vi "TEST_MenuRTM.vi"(10 "Color Theme":enum16{"LabVIEW", "Dark", "Windows Gray"}(ring), 11 "ExitEvent":refnum<user-event>) -> ()   [LabVIEW 2021]
uses:
  Menu.lvclass
  Picture2D/src/Font/Font.lvclass
  Picture2D/src/Square/Square.lvclass
  C:/GitHub/Picture2D/src/Polygone/Polygone.lvclass
  C:/GitHub/Picture2D/src/Rectangle/Rectangle.lvclass
  C:/GitHub/Picture2D/src/Shape/Shape.lvclass
  C:/GitHub/Picture2D/src/Picture2D/Picture2D.lvclass
  Picture2D/src/Point/Point.lvclass
  Picture2D/src/Font/Font.lvclass/Font.ctl
  Picture2D/src/Color/Color.lvclass
  SubMenuIcon.ctl
  4d7882bf-4570-41b5-8159-e9b7f331f501.vi
  Picture2D/src/Font/SetFontName.vi
  Picture2D/src/Font/SetSize.vi
  SetBackgroundColor.vi
  SetBorderColor.vi
  SetHiliteColor.vi
  SetHiliteTextColor.vi
  SetTextColor.vi
  SetFont.vi
  SetDesiredFont.vi
  SetSubMenuIconType.vi
  SetSubMenuIconOpened.vi
  SetSubMenuIconClosed.vi
  <vilib>/ErrorRing/Error Ring.xnode
panel:
  out "2D Picture":picture
  in  "Font Name":string="Arial"
  in  "Size":i16=16
  in  "Desired Font":T1(ring)=enum."Application Font"
  out "ItemPath":string
  out "ItemTag":string
  out "error out":errorcluster
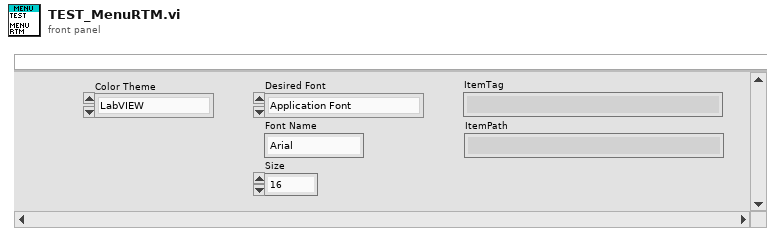
[diagram p1: front panel]
types:
  T1 = enum16{"User-specified Font", "Application Font", "System Font", "Dialog Font"}
  T2 = typedef "Menu.lvlib/Menu.lvclass/SubMenuIcon.ctl" = enum16{"LabVIEW", "Windows", "Custom"}
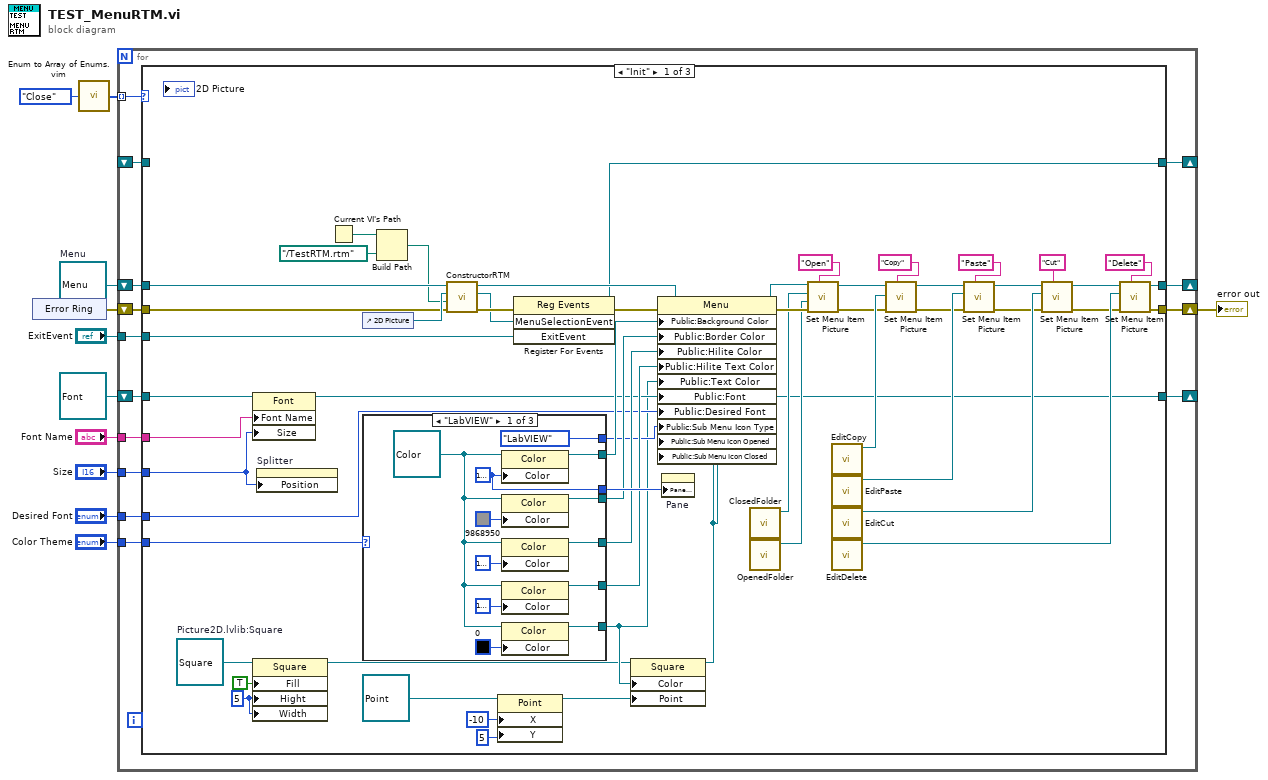
[diagram p0: block diagram]
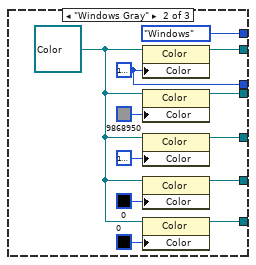
[diagram p2: hidden frame]
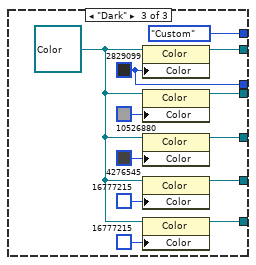
[diagram p3: hidden frame]
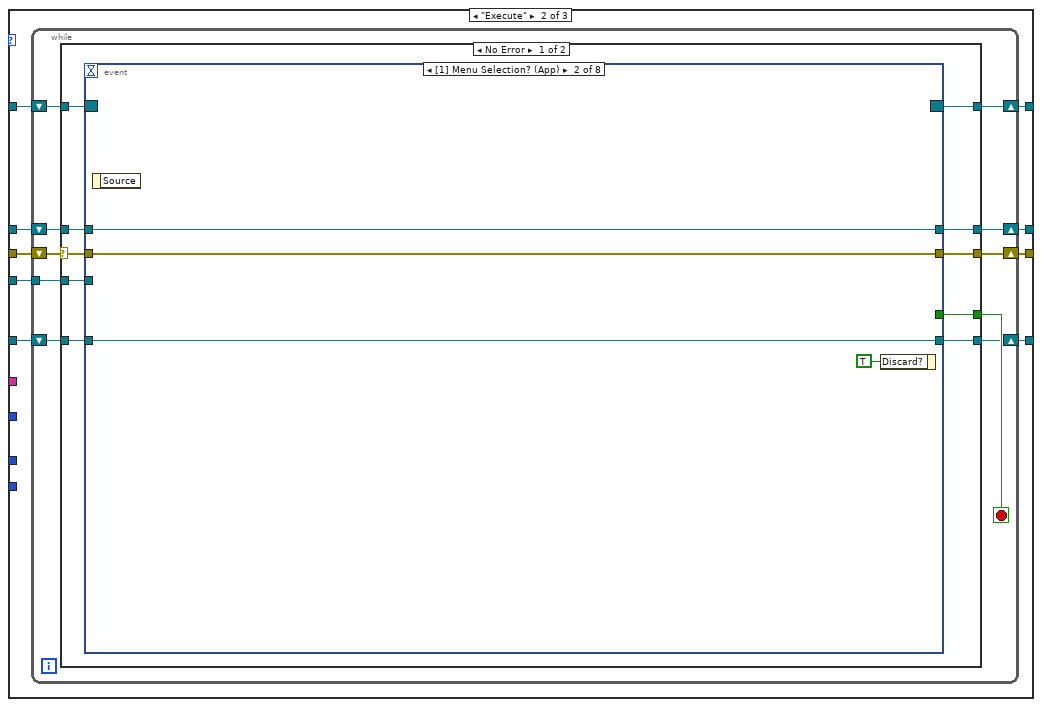
[diagram p4: hidden frame]
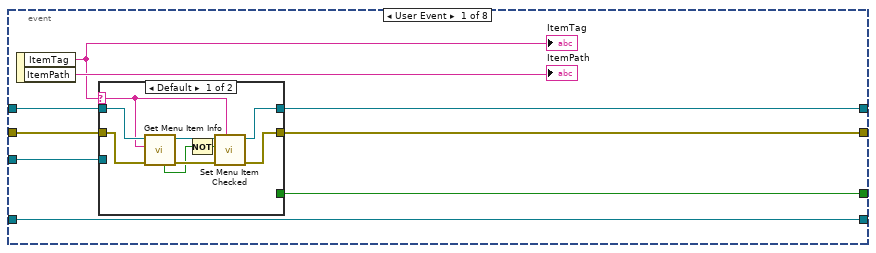
[diagram p5: hidden frame]
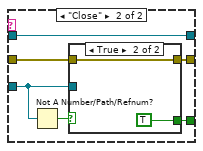
[diagram p6: hidden frame]
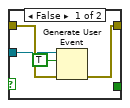
[diagram p7: hidden frame]
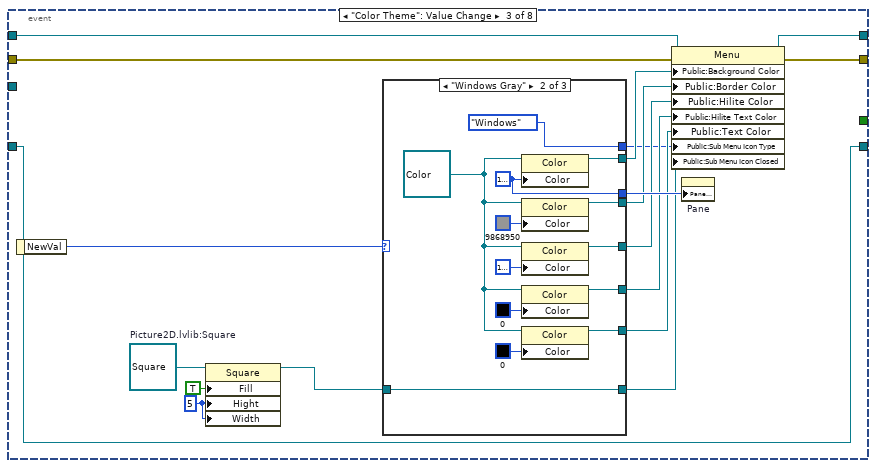
[diagram p8: hidden frame]
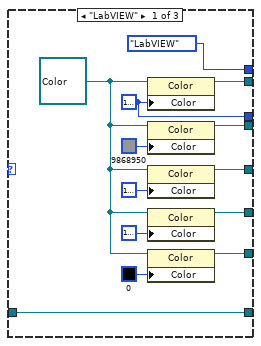
[diagram p9: hidden frame]
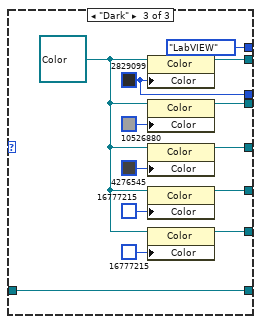
[diagram p10: hidden frame]
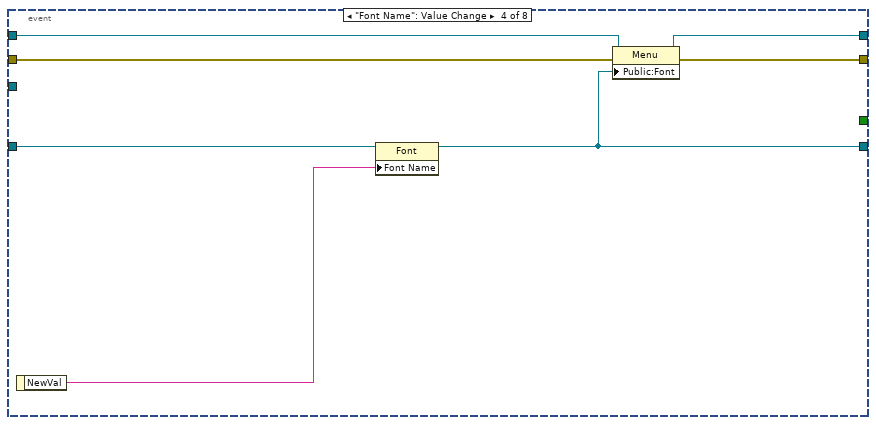
[diagram p11: hidden frame]
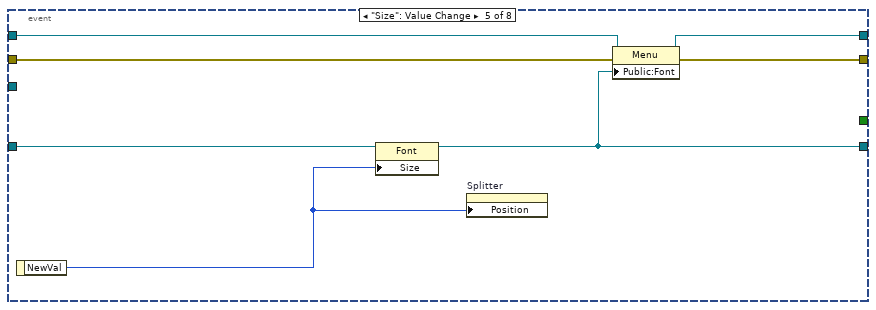
[diagram p12: hidden frame]
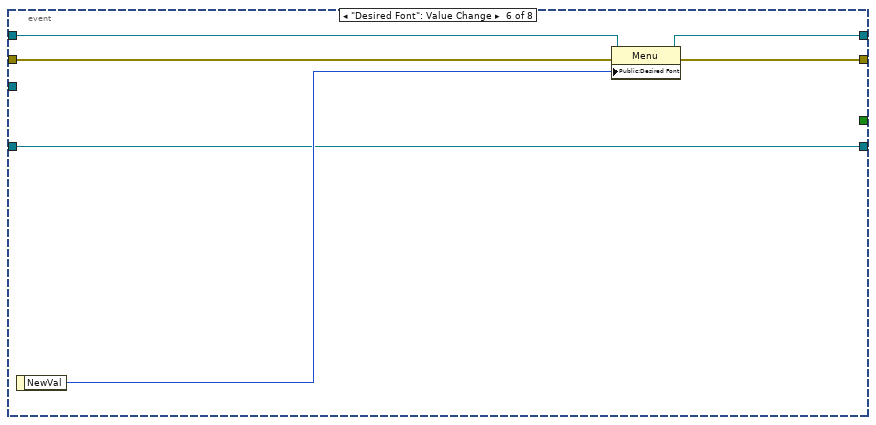
[diagram p13: hidden frame]
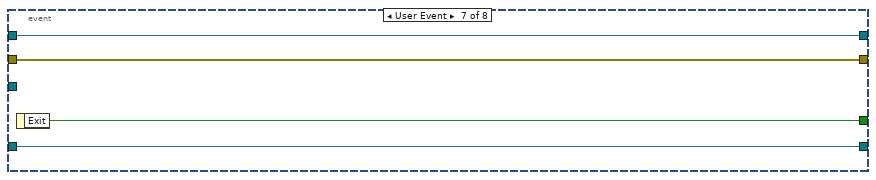
[diagram p14: hidden frame]
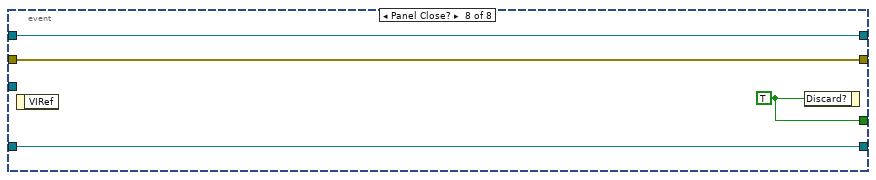
[diagram p15: hidden frame]
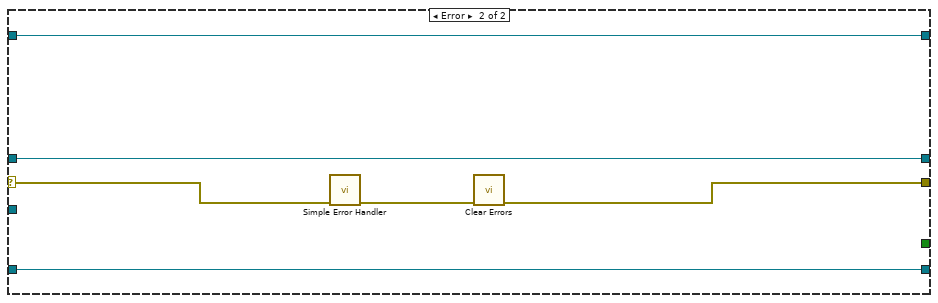
[diagram p16: hidden frame]
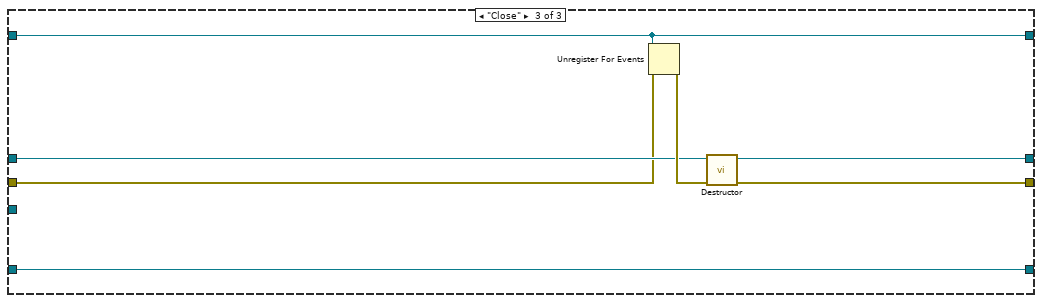
[diagram p17: hidden frame]
diagram:
  w3 = refnum<class "Menu.lvclass"> refnum  # Menu
  n1 = xnode "Error Ring"() -> ("error out"=w2:errorcluster)
  n2 = call "Enum to Array of Enums.vim"("enum"=enum16{"Init", "Execute", "Close"}."Close") -> ("array of enums"=w10:enum16{"Init", "Execute", "Close"}[])
  n3 = for {
    tunnel: "ExitEvent" -> [w22]
    shift-right: [w12] -> _
    shift-left: _ -> [w25]
    shift-right: [w14] -> w1
    shift-left: w2 -> [w24]
    shift-right: [w13] -> _
    shift-left: w3 -> [w23]
    tunnel: w10 -> [w21] mode=indexing
    tunnel: "Font Name" -> [w19]
    tunnel: "Size" -> [w18]
    tunnel: "Desired Font" -> [w17]
    tunnel: "Color Theme" -> [w16]
    shift-right: [w15] -> _
    shift-left: refnum<class "Font.lvclass"> refnum ("Fonts") -> [w20]
    n4 = case shown="\"Init\"" w21 {
      tunnel: w25 -> [_ w127 w274]
      tunnel: [w46 w126 w275] -> w13
      tunnel: [w44 w125 w274] -> w12
      tunnel: [w45 w124 w277] -> w14
      tunnel: w24 -> [w38 w123 w273]
      tunnel: w23 -> [w47 w122 w275]
      tunnel: w22 -> [w43 w121 _]
      tunnel: w20 -> [w56 w120 w276]
      tunnel: w19 -> [w55 _ _]
      tunnel: w18 -> [w37 _ _]
      tunnel: w17 -> [w54 _ _]
      tunnel: w16 -> [w48 _ _]
      tunnel: [w42 w119 w276] -> w15
      frame "Init" {
        w33 = i16 5 ("Hight")
        w35 = refnum<class "Square.lvclass"> refnum  # Picture2D.lvlib:Square
        n5 = property class="Font"(reference=w56, "Font Name"=w55, "Size"=w37) -> (reference out=w42:refnum<class "Font.lvclass">)  [unwired: 1 in, 1 out]
        n6 = property class="Square"(reference=w35, "Fill"=TRUE, "Hight"=w33, "Width"=w33) -> (reference out=w27:refnum<class "Square.lvclass">)  [unwired: 1 in, 1 out]
        n7 = property on="Splitter" class="Splitter"("Position"=w37) -> ()  [unwired: 2 in, 2 out]
        n8 = Current VI's Path() -> (path=w41:path)
        n9 = control-ref of="2D Picture"() -> (w60:refnum<vi>)
        n10 = case shown="\"LabVIEW\"" w48 {
          tunnel: [w94 w106 w118] -> w62
          tunnel: [w92 w104 w116] -> w63
          tunnel: [w91 w103 w115] -> w64
          tunnel: [w90 w102 w114] -> w65
          tunnel: [w89 w101 w113] -> w32
          tunnel: [w84 w96 w108] -> w66
          tunnel: [SubMenuIcon."LabVIEW" ("SubMenuIconType") SubMenuIcon."Windows" ("SubMenuIconType") SubMenuIcon."Custom" ("SubMenuIconType")] -> w36
          frame "LabVIEW" {
            w84 = u32 16777238 ("Color")
            w93 = refnum<class "Color.lvclass"> refnum ("Background Color")
            n11 = property class="Color"(reference=w93, "Color"=w84) -> (reference out=w94:refnum<class "Color.lvclass">)  [unwired: 1 in, 1 out]
            n12 = property class="Color"(reference=w93, "Color"=u32 9868950) -> (reference out=w92:refnum<class "Color.lvclass">)  [unwired: 1 in, 1 out]
            n13 = property class="Color"(reference=w93, "Color"=u32 16777224) -> (reference out=w91:refnum<class "Color.lvclass">)  [unwired: 1 in, 1 out]
            n14 = property class="Color"(reference=w93, "Color"=u32 16777226) -> (reference out=w90:refnum<class "Color.lvclass">)  [unwired: 1 in, 1 out]
            n15 = property class="Color"(reference=w93, "Color"=u32 0) -> (reference out=w89:refnum<class "Color.lvclass">)  [unwired: 1 in, 1 out]
          }
          frame "Windows Gray" {
            w96 = u32 16777238 ("Color")
            w105 = refnum<class "Color.lvclass"> refnum ("Background Color")
            n16 = property class="Color"(reference=w105, "Color"=w96) -> (reference out=w106:refnum<class "Color.lvclass">)  [unwired: 1 in, 1 out]
            n17 = property class="Color"(reference=w105, "Color"=u32 9868950) -> (reference out=w104:refnum<class "Color.lvclass">)  [unwired: 1 in, 1 out]
            n18 = property class="Color"(reference=w105, "Color"=u32 16777225) -> (reference out=w103:refnum<class "Color.lvclass">)  [unwired: 1 in, 1 out]
            n19 = property class="Color"(reference=w105, "Color"=u32 0) -> (reference out=w102:refnum<class "Color.lvclass">)  [unwired: 1 in, 1 out]
            n20 = property class="Color"(reference=w105, "Color"=u32 0) -> (reference out=w101:refnum<class "Color.lvclass">)  [unwired: 1 in, 1 out]
          }
          frame "Dark" {
            w108 = u32 2829099 ("Color")
            w117 = refnum<class "Color.lvclass"> refnum ("Background Color")
            n21 = property class="Color"(reference=w117, "Color"=w108) -> (reference out=w118:refnum<class "Color.lvclass">)  [unwired: 1 in, 1 out]
            n22 = property class="Color"(reference=w117, "Color"=u32 10526880) -> (reference out=w116:refnum<class "Color.lvclass">)  [unwired: 1 in, 1 out]
            n23 = property class="Color"(reference=w117, "Color"=u32 4276545) -> (reference out=w115:refnum<class "Color.lvclass">)  [unwired: 1 in, 1 out]
            n24 = property class="Color"(reference=w117, "Color"=u32 16777215) -> (reference out=w114:refnum<class "Color.lvclass">)  [unwired: 1 in, 1 out]
            n25 = property class="Color"(reference=w117, "Color"=u32 16777215) -> (reference out=w113:refnum<class "Color.lvclass">)  [unwired: 1 in, 1 out]
          }
        }
        n26 = Build Path(base path=w41, name or relative path=path "../TestRTM.rtm") -> (appended path=w39:path)
        n27 = call "ConstructorRTM.vi"("error in (no error)"=w38, "RTM Path"=w39, "PictRef"=w60, "Menu in"=w47) -> ("error out"=w59:errorcluster, "MenuSelectionEvent"=w57:refnum<user-event>, "Menu out"=w61:refnum<class "Menu.lvclass">)  [unwired: 5 in]
        n28 = property class="Point"(reference=refnum<class "Point.lvclass"> refnum ("Point"), "X"=i16 -10, "Y"=i16 5) -> (reference out=w30:refnum<class "Point.lvclass">)  [unwired: 1 in, 1 out]
        n29 = register-events(error in=w59, w57, w43) -> (reference out=w44:refnum<event-registration>, error out=w58:errorcluster)  [unwired: 1 in]
        n30 = property class="Square"(reference=w27, "Color"=w32, "Point"=w30) -> (reference out=w26:refnum<class "Square.lvclass">)  [unwired: 1 in, 1 out]
        n31 = property class="Menu"(reference=w61, error in=w58, "Public:Background Color"=w62, "Public:Border Color"=w63, "Public:Hilite Color"=w64, "Public:Hilite Text Color"=w65, "Public:Text Color"=w32, "Public:Font"=w42, "Public:Desired Font"=w54, "Public:Sub Menu Icon Type"=w36, "Public:Sub Menu Icon Opened"=w26, "Public:Sub Menu Icon Closed"=w26) -> (reference out=w81:refnum<class "Menu.lvclass">, error out=w82:errorcluster)
        n32 = property on="Pane" class="Pane"("PaneColor"=w66) -> ()  [unwired: 2 in, 2 out]
        n33 = call "ClosedFolder.vi"() -> ("Image out"=w79:refnum<class "Image.lvclass">)  [unwired: 11 in]
        n34 = call "OpenedFolder.vi"() -> ("Image out"=w80:refnum<class "Image.lvclass">)  [unwired: 11 in]
        n35 = call "Set Menu Item Picture.vi"("item tag"="Open", "error in (no error)"=w82, "Hilite Picture"=w80, "Picture"=w79, "Menu in"=w81) -> ("error out"=w68:errorcluster, "Menu out"=w67:refnum<class "Menu.lvclass">)  [unwired: 5 in]
        n36 = call "EditCopy.vi"() -> ("Image out"=w75:refnum<class "Image.lvclass">)  [unwired: 11 in]
        n37 = call "EditPaste.vi"() -> ("Image out"=w76:refnum<class "Image.lvclass">)  [unwired: 11 in]
        n38 = call "EditCut.vi"() -> ("Image out"=w77:refnum<class "Image.lvclass">)  [unwired: 11 in]
        n39 = call "EditDelete.vi"() -> ("Image out"=w78:refnum<class "Image.lvclass">)  [unwired: 11 in]
        n40 = call "Set Menu Item Picture.vi"("item tag"="Copy", "error in (no error)"=w68, "Picture"=w75, "Menu in"=w67) -> ("error out"=w70:errorcluster, "Menu out"=w69:refnum<class "Menu.lvclass">)  [unwired: 6 in]
        n41 = call "Set Menu Item Picture.vi"("item tag"="Paste", "error in (no error)"=w70, "Picture"=w76, "Menu in"=w69) -> ("error out"=w72:errorcluster, "Menu out"=w71:refnum<class "Menu.lvclass">)  [unwired: 6 in]
        n42 = call "Set Menu Item Picture.vi"("item tag"="Cut", "error in (no error)"=w72, "Picture"=w77, "Menu in"=w71) -> ("error out"=w74:errorcluster, "Menu out"=w73:refnum<class "Menu.lvclass">)  [unwired: 6 in]
        n43 = call "Set Menu Item Picture.vi"("item tag"="Delete", "error in (no error)"=w74, "Picture"=w78, "Menu in"=w73) -> ("error out"=w45:errorcluster, "Menu out"=w46:refnum<class "Menu.lvclass">)  [unwired: 6 in]
      }
      frame "Execute" {
        n44 = while {
          shift-right: [w135] -> w124
          shift-left: w123 -> [w136]
          shift-right: [w132] -> w125
          shift-left: w127 -> [w137]
          shift-right: [w133] -> w126
          shift-left: w122 -> [w134]
          tunnel: w121 -> [w130]
          shift-right: [w128] -> w119
          shift-left: w120 -> [w129]
          stop <- w131 stop-if-true
          n45 = case shown="No Error" w136 {
            selector: w136 -> [w146 w272]
            tunnel: w137 -> [w147 w271]
            tunnel: [w145 w268] -> w135
            tunnel: w134 -> [w144 w270]
            tunnel: [w143 w270] -> w133
            tunnel: [w142 w271] -> w132
            tunnel: [w141 _] -> w131
            tunnel: w130 -> [w140 _]
            tunnel: w129 -> [w139 w267]
            tunnel: [w138 w267] -> w128
            frame No Error {
              n46 = event shown="[1] Menu Selection? (App)" {
                selector: w147 -> [_ _ _ _ _ _ _ _]
                dyn-events: [_ _ _ _ _ _ _ _] -> w142
                timeout: _ -> [_ _ _ _ _ _ _ _]
                tunnel: [w153 w181 w192 w242 w250 w258 w262 w265] -> w145
                tunnel: w146 -> [w154 w181 w193 w241 w249 w257 w262 w265]
                tunnel: [w152 w180 w191 w240 w248 w256 w261 w264] -> w143
                tunnel: w144 -> [w155 w180 w190 w239 w247 w255 w261 w264]
                tunnel: [w150 _ _ _ _ _ w260 w266] -> w141
                tunnel: w140 -> [w151 _ _ _ _ _ _ _]
                tunnel: w139 -> [w149 w179 w188 w245 w252 w253 w259 w263]
                tunnel: [w149 w179 w188 w244 w251 w253 w259 w263] -> w138
                event User Event {
                  n47 = event-data() -> ("ItemTag"=w148:string, "ItemPath"=→"ItemPath":string)  [unwired: 1 in]
                  "ItemTag" <- w148
                  n48 = case shown="Default" w148 {
                    selector: w148 -> [w157 _]
                    tunnel: w155 -> [w165 w171]
                    tunnel: w154 -> [w164 w169]
                    tunnel: [w162 w170] -> w153
                    tunnel: [w160 w171] -> w152
                    tunnel: w151 -> [_ w168]
                    tunnel: [_ w166] -> w150
                    frame Default {
                      n49 = call "Get Menu Item Info.vi"("error in (no error)"=w164, "item tag"=w157, "Menu in"=w165) -> ("error out"=w163:errorcluster, "Menu out"=w161:refnum<class "Menu.lvclass">, "checked"=w159:bool)  [unwired: 1 in, 5 out]
                      n50 = Not(x=w159) -> (.not. x?=w158:bool)
                      n51 = call "Set Menu Item Checked.vi"("item tag"=w157, "error in (no error)"=w163, "checked"=w158, "Menu in"=w161) -> ("error out"=w162:errorcluster, "Menu out"=w160:refnum<class "Menu.lvclass">)  [unwired: 6 in]
                    }
                    frame "Close" {
                      n52 = Not A Number/Path/Refnum?(number/path/refnum=w168) -> (NaN/Path/Refnum?=w167:bool)
                      n53 = case shown="True" w167 {
                        tunnel: [w175 w177] -> w170
                        tunnel: w169 -> [w174 w177]
                        tunnel: w168 -> [w172 _]
                        tunnel: [_ TRUE] -> w166
                        frame False {
                          n54 = Generate User Event(user event=w172, event data cluster=TRUE ("event data"), error in=w174) -> (error out=w175:errorcluster)  [unwired: 1 in, 1 out]
                        }
                        frame True {
                        }
                      }
                    }
                  }
                }
                event Menu Selection? (App) {
                  n55 = event-data() -> ()  [unwired: 1 in, 1 out]
                  n56 = event-data("Discard?"=TRUE) -> ()  [unwired: 1 in, 1 out]
                }
                event "Color Theme": Value Change {
                  w184 = i16 5 ("Hight")
                  w186 = refnum<class "Square.lvclass"> refnum  # Picture2D.lvlib:Square
                  n57 = event-data() -> ("NewVal"=w189:enum16{"LabVIEW", "Dark", "Windows Gray"})  [unwired: 1 in]
                  n58 = property class="Square"(reference=w186, "Fill"=TRUE, "Hight"=w184, "Width"=w184) -> (reference out=w183:refnum<class "Square.lvclass">)  [unwired: 1 in, 1 out]
                  n59 = case shown="\"Windows Gray\"" w189 {
                    tunnel: [w212 w225 w238] -> w194
                    tunnel: [w210 w223 w236] -> w195
                    tunnel: [w209 w222 w235] -> w196
                    tunnel: [w208 w221 w234] -> w197
                    tunnel: [w207 w220 w233] -> w198
                    tunnel: [w202 w215 w228] -> w199
                    tunnel: [SubMenuIcon."LabVIEW" ("SubMenuIconType") SubMenuIcon."Windows" ("SubMenuIconType") SubMenuIcon."LabVIEW" ("SubMenuIconType")] -> w187
                    tunnel: [w200 w213 w226] -> w182
                    tunnel: w183 -> [w200 w213 w226]
                    frame "LabVIEW" {
                      w202 = u32 16777238 ("Color")
                      w211 = refnum<class "Color.lvclass"> refnum ("Background Color")
                      n60 = property class="Color"(reference=w211, "Color"=w202) -> (reference out=w212:refnum<class "Color.lvclass">)  [unwired: 1 in, 1 out]
                      n61 = property class="Color"(reference=w211, "Color"=u32 9868950) -> (reference out=w210:refnum<class "Color.lvclass">)  [unwired: 1 in, 1 out]
                      n62 = property class="Color"(reference=w211, "Color"=u32 16777224) -> (reference out=w209:refnum<class "Color.lvclass">)  [unwired: 1 in, 1 out]
                      n63 = property class="Color"(reference=w211, "Color"=u32 16777226) -> (reference out=w208:refnum<class "Color.lvclass">)  [unwired: 1 in, 1 out]
                      n64 = property class="Color"(reference=w211, "Color"=u32 0) -> (reference out=w207:refnum<class "Color.lvclass">)  [unwired: 1 in, 1 out]
                    }
                    frame "Windows Gray" {
                      w215 = u32 16777238 ("Color")
                      w224 = refnum<class "Color.lvclass"> refnum ("Background Color")
                      n65 = property class="Color"(reference=w224, "Color"=w215) -> (reference out=w225:refnum<class "Color.lvclass">)  [unwired: 1 in, 1 out]
                      n66 = property class="Color"(reference=w224, "Color"=u32 9868950) -> (reference out=w223:refnum<class "Color.lvclass">)  [unwired: 1 in, 1 out]
                      n67 = property class="Color"(reference=w224, "Color"=u32 16777225) -> (reference out=w222:refnum<class "Color.lvclass">)  [unwired: 1 in, 1 out]
                      n68 = property class="Color"(reference=w224, "Color"=u32 0) -> (reference out=w221:refnum<class "Color.lvclass">)  [unwired: 1 in, 1 out]
                      n69 = property class="Color"(reference=w224, "Color"=u32 0) -> (reference out=w220:refnum<class "Color.lvclass">)  [unwired: 1 in, 1 out]
                    }
                    frame "Dark" {
                      w228 = u32 2829099 ("Color")
                      w237 = refnum<class "Color.lvclass"> refnum ("Background Color")
                      n70 = property class="Color"(reference=w237, "Color"=w228) -> (reference out=w238:refnum<class "Color.lvclass">)  [unwired: 1 in, 1 out]
                      n71 = property class="Color"(reference=w237, "Color"=u32 10526880) -> (reference out=w236:refnum<class "Color.lvclass">)  [unwired: 1 in, 1 out]
                      n72 = property class="Color"(reference=w237, "Color"=u32 4276545) -> (reference out=w235:refnum<class "Color.lvclass">)  [unwired: 1 in, 1 out]
                      n73 = property class="Color"(reference=w237, "Color"=u32 16777215) -> (reference out=w234:refnum<class "Color.lvclass">)  [unwired: 1 in, 1 out]
                      n74 = property class="Color"(reference=w237, "Color"=u32 16777215) -> (reference out=w233:refnum<class "Color.lvclass">)  [unwired: 1 in, 1 out]
                    }
                  }
                  n75 = property class="Menu"(reference=w190, error in=w193, "Public:Background Color"=w194, "Public:Border Color"=w195, "Public:Hilite Color"=w196, "Public:Hilite Text Color"=w197, "Public:Text Color"=w198, "Public:Sub Menu Icon Type"=w187, "Public:Sub Menu Icon Closed"=w182) -> (reference out=w191:refnum<class "Menu.lvclass">, error out=w192:errorcluster)
                  n76 = property on="Pane" class="Pane"("PaneColor"=w199) -> ()  [unwired: 2 in, 2 out]
                }
                event "Font Name": Value Change {
                  n77 = event-data() -> ("NewVal"=w243:string)  [unwired: 1 in]
                  n78 = property class="Font"(reference=w245, "Font Name"=w243) -> (reference out=w244:refnum<class "Font.lvclass">)  [unwired: 1 in, 1 out]
                  n79 = property class="Menu"(reference=w239, error in=w241, "Public:Font"=w244) -> (reference out=w240:refnum<class "Menu.lvclass">, error out=w242:errorcluster)
                }
                event "Size": Value Change {
                  n80 = event-data() -> ("NewVal"=w246:i16)  [unwired: 1 in]
                  n81 = property class="Font"(reference=w252, "Size"=w246) -> (reference out=w251:refnum<class "Font.lvclass">)  [unwired: 1 in, 1 out]
                  n82 = property on="Splitter" class="Splitter"("Position"=w246) -> ()  [unwired: 2 in, 2 out]
                  n83 = property class="Menu"(reference=w247, error in=w249, "Public:Font"=w251) -> (reference out=w248:refnum<class "Menu.lvclass">, error out=w250:errorcluster)
                }
                event "Desired Font": Value Change {
                  n84 = event-data() -> ("NewVal"=w254:T1)  [unwired: 1 in]
                  n85 = property class="Menu"(reference=w255, error in=w257, "Public:Desired Font"=w254) -> (reference out=w256:refnum<class "Menu.lvclass">, error out=w258:errorcluster)
                }
                event User Event {
                  n86 = event-data() -> ("Exit"=w260:bool)  [unwired: 1 in]
                }
                event Panel Close? {
                  w266 = TRUE ("Discard?")
                  n87 = event-data() -> ()  [unwired: 1 in, 1 out]
                  n88 = event-data("Discard?"=w266) -> ()  [unwired: 1 in, 1 out]
                }
              }
            }
            frame Error {
              n89 = call <vilib>:"Simple Error Handler.vi"("error in (no error)"=w272) -> ("error out"=w269:errorcluster)  [unwired: 4 in, 4 out]
              n90 = call <vilib>:"Clear Errors.vi"("error in (no error)"=w269) -> ("error out"=w268:errorcluster)  [unwired: 5 in, 1 out]
            }
          }
        }
      }
      frame "Close" {
        n91 = Unregister For Events(event registration refnum=w274, error in=w273) -> (error out=w278:errorcluster)
        n92 = call "Destructor.vi"("error in (no error)"=w278, "Menu in"=w275) -> ("error out"=w277:errorcluster)  [unwired: 9 in]
      }
    }
  }
  "error out" <- w1
